vi "Handle Command.vi"(8 "error in (no error)":errorcluster, 9 "Data":variant, 10 "Command":string, 11 "RP100 in":refnum<class "RP100.lvclass">) -> (0 "error out":errorcluster, 1 "Processed Data":variant, 2 "Command":string, 3 "RP100 out":refnum<class "RP100.lvclass">)   [LabVIEW 2019, in "RP100.lvclass"]
uses:
  RP100.lvclass
  Typedefs/Output Channel--Enum.ctl
  Typedefs/Output State--Enum.ctl
  Typedefs/setStrain--Cluster.ctl
  RP100.lvclass/RP100.ctl
  Typedefs/setOutput--Cluster.ctl
  Typedefs/setLevel--Cluster.ctl
  Typedefs/getLevel--Cluster.ctl
  144ac86c-f3d3-4b89-933e-c91cd0042f1d.vi
  aaf9e925-0147-4d55-b975-571e4f63da02.vi
  6c0bf34a-ab55-4634-99ae-1a4930a83075.vi
  8b117c61-ef82-475d-98ae-2b78dab96990.vi
  <vilib>/JDP Science/JSONtext/JSON text to Variant.vi
  <vilib>/JDP Science/JSONtext/LVClass Serializer/JSONtext LVClass Serializer.lvclass
  <userlib>/LevyLab/Instrument Framework/Instrument Types/Strain/Instrument.Strain.lvclass
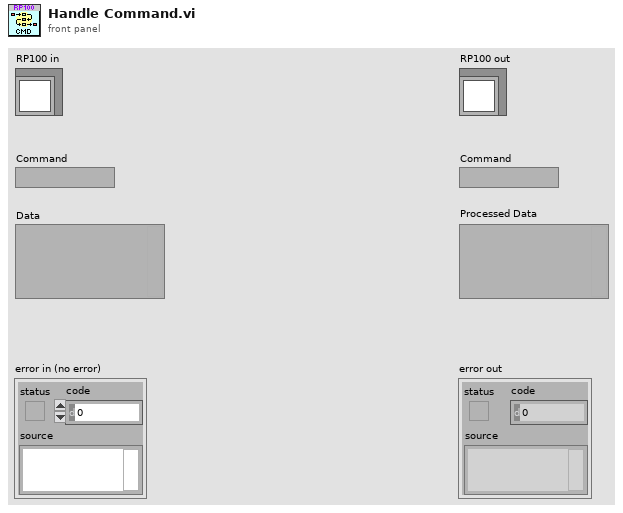
[diagram p1: front panel]
types:
  T1 = typedef "RP100.lvclass/setStrain--Cluster.ctl" = cluster{"Strain (V)":dbl, "Slew (V/s)":dbl}
  T2 = typedef "RP100.lvclass/Output Channel--Enum.ctl" = enum16{"Output 1", "Output 2"}
  T3 = typedef "RP100.lvclass/Output State--Enum.ctl" = enum16{"Shorted", "Enabled"}
  T4 = typedef "RP100.lvclass/setOutput--Cluster.ctl" = cluster{"State":T3}
  T5 = typedef "RP100.lvclass/setLevel--Cluster.ctl" = cluster{"Output Channel":T2, "Level (V)":dbl, "Slew (V/s)":dbl}
  T6 = typedef "RP100.lvclass/getLevel--Cluster.ctl" = cluster{"Channel":T2}
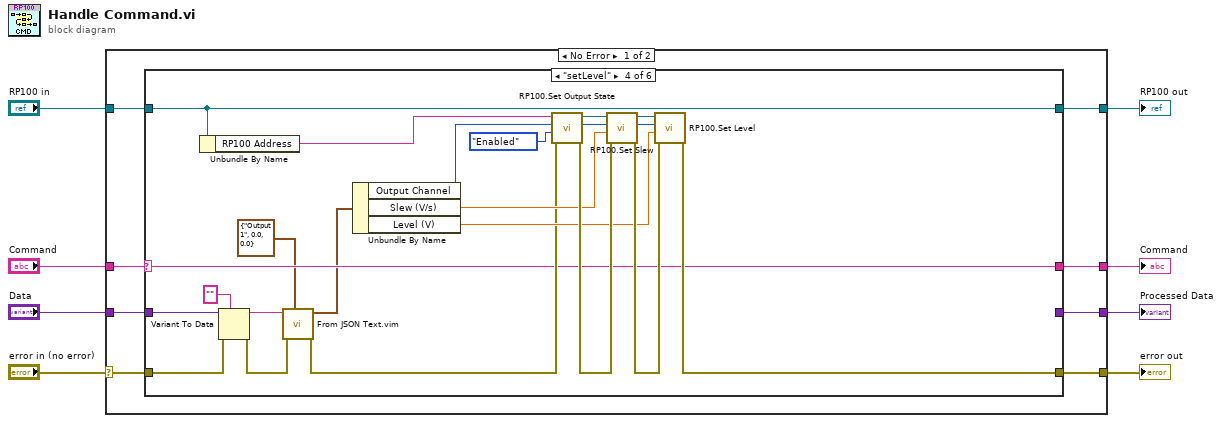
[diagram p0: block diagram]
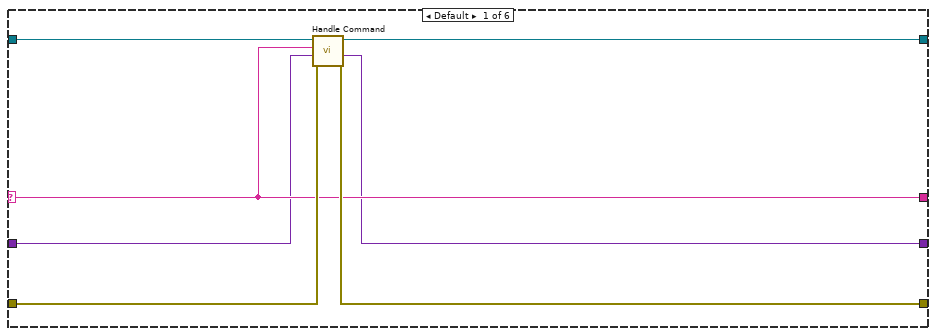
[diagram p2: hidden frame]
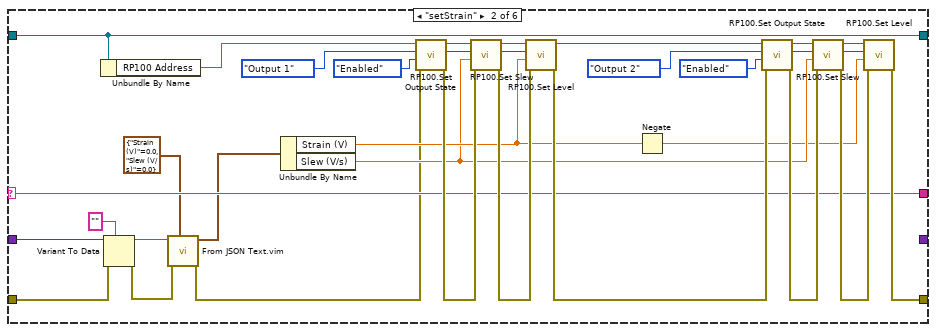
[diagram p3: hidden frame]
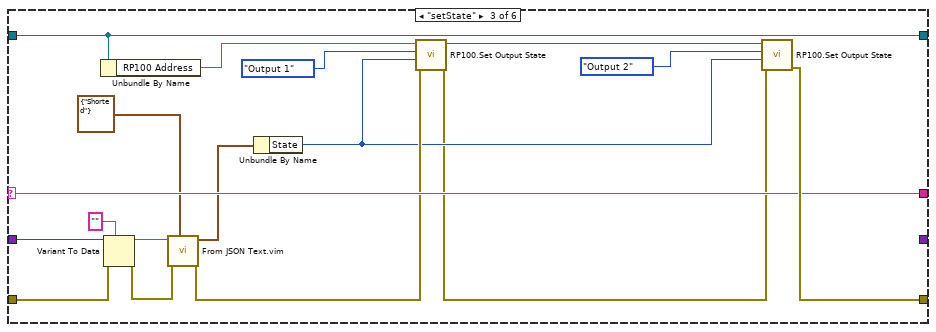
[diagram p4: hidden frame]
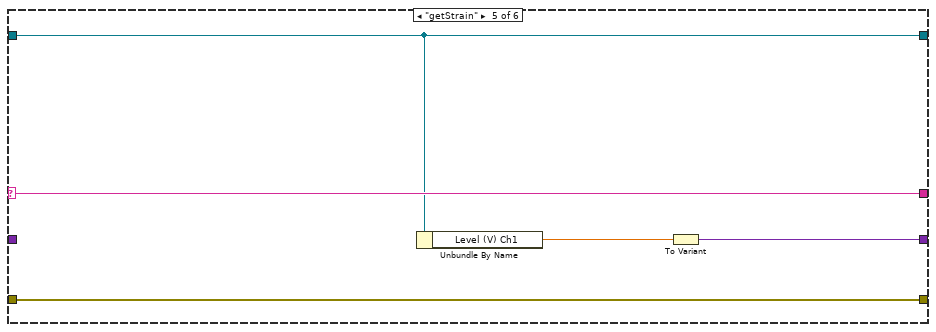
[diagram p5: hidden frame]
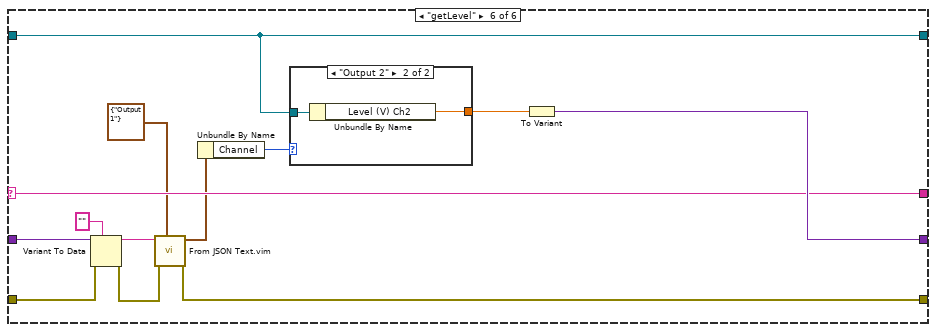
[diagram p6: hidden frame]
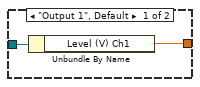
[diagram p7: hidden frame]
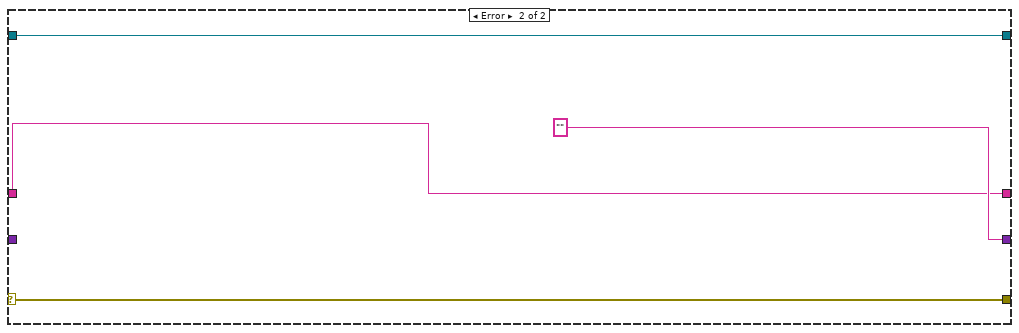
[diagram p8: hidden frame]
diagram:
  n1 = case shown="No Error" "error in (no error)" {
    selector: "error in (no error)" -> [w13 w121]
    tunnel: [w12 w121] -> w4
    tunnel: [w15 w120] -> w6
    tunnel: "RP100 in" -> [w16 w120]
    tunnel: "Command" -> [w10 w118]
    tunnel: [w14 "" ("error message (\"\")")] -> w3
    tunnel: [w11 w118] -> w2
    tunnel: "Data" -> [w9 _]
    frame No Error {
      n2 = case shown="\"setLevel\"" w10 {
        selector: w10 -> [w21 w35 w70 w80 w99 w109]
        tunnel: w16 -> [w20 w27 w64 w76 w96 w111]
        tunnel: [w19 w27 w64 w76 w96 w111] -> w15
        tunnel: [w17 _ _ _ w98 w113] -> w14
        tunnel: w13 -> [w23 w26 w63 w75 w100 w106]
        tunnel: [w22 w48 w71 w92 w100 w104] -> w12
        tunnel: [w21 w35 w70 w80 w99 w109] -> w11
        tunnel: w9 -> [w18 w32 w67 w82 _ w108]
        frame Default {
          n3 = call-parent "Handle Command.vi"("error in (no error)"=w23, "Data"=w18, "Command"=w21, "Instrument in"=w20) -> ("error out"=w22:errorcluster, "Processed Data"=w17:variant, "Instrument out"=w19:refnum<class "RP100.lvclass">)  [unwired: 4 in, 1 out]
        }
        frame "setStrain" {
          n4 = Unbundle By Name(w27) -> ("RP100 Address"=w25:string)
          n5 = Variant To Data(error in=w26, type="", Variant=w32) -> (data=w34:string, error out=w31:errorcluster)
          n6 = call "From JSON Text.vim"("Data Type and Default Value"=T1 {"Strain (V)"=0.0, "Slew (V/s)"=0.0} ("setStrain"), "error in (no error)"=w31, "JSON"=w34) -> ("error out"=w30:errorcluster, "Data out"=w24:T1)  [unwired: 7 in]
          n7 = Unbundle By Name(w24) -> ("Strain (V)"=w47:dbl, "Slew (V/s)"=w40:dbl)
          n8 = call "RP100.Set Output State.vi"("error in (no error)"=w30, "Output State"=Output_State--Enum."Enabled", "Output Channel"=Output_Channel--Enum."Output 1", "VISA resource name"=w25) -> ("error out"=w53:errorcluster, "Output Channel"=w45:T2, "VISA Refnum out"=w46:refnum<visa-resource-name>)  [unwired: 5 in]
          n9 = call "RP100.Set Slew.vi"("error in (no error)"=w53, "Slew (V/s)"=w40, "Output Channel"=w45, "VISA resource name"=w46) -> ("error out"=w52:errorcluster, "Output Channel"=w44:T2, "VISA Refnum out"=w43:refnum<visa-resource-name>)  [unwired: 5 in]
          n10 = call "RP100.Set Level.vi"("error in (no error)"=w52, "Level (V)"=w47, "Output Channel"=w44, "VISA resource name"=w43) -> ("error out"=w51:errorcluster, "VISA Refnum out"=w42:refnum<visa-resource-name>)  [unwired: 5 in, 1 out]
          n11 = Negate(x=w47) -> (-x=w39:dbl)
          n12 = call "RP100.Set Output State.vi"("error in (no error)"=w51, "Output State"=Output_State--Enum."Enabled", "Output Channel"=Output_Channel--Enum."Output 2", "VISA resource name"=w42) -> ("error out"=w50:errorcluster, "Output Channel"=w41:T2, "VISA Refnum out"=w36:refnum<visa-resource-name>)  [unwired: 5 in]
          n13 = call "RP100.Set Slew.vi"("error in (no error)"=w50, "Slew (V/s)"=w40, "Output Channel"=w41, "VISA resource name"=w36) -> ("error out"=w49:errorcluster, "Output Channel"=w38:T2, "VISA Refnum out"=w37:refnum<visa-resource-name>)  [unwired: 5 in]
          n14 = call "RP100.Set Level.vi"("error in (no error)"=w49, "Level (V)"=w39, "Output Channel"=w38, "VISA resource name"=w37) -> ("error out"=w48:errorcluster)  [unwired: 5 in, 2 out]
        }
        frame "setState" {
          n15 = Unbundle By Name(w64) -> ("RP100 Address"=w62:string)
          n16 = Variant To Data(error in=w63, type="", Variant=w67) -> (data=w69:string, error out=w66:errorcluster)
          n17 = call "From JSON Text.vim"("Data Type and Default Value"=T4 {"State"=enum."Shorted"} ("setOutput"), "error in (no error)"=w66, "JSON"=w69) -> ("error out"=w65:errorcluster, "Data out"=w61:T4)  [unwired: 7 in]
          n18 = Unbundle By Name(w61) -> ("State"=w59:T3)
          n19 = call "RP100.Set Output State.vi"("error in (no error)"=w65, "Output State"=w59, "Output Channel"=Output_Channel--Enum."Output 1", "VISA resource name"=w62) -> ("error out"=w57:errorcluster, "VISA Refnum out"=w58:refnum<visa-resource-name>)  [unwired: 5 in, 1 out]
          n20 = call "RP100.Set Output State.vi"("error in (no error)"=w57, "Output State"=w59, "Output Channel"=Output_Channel--Enum."Output 2", "VISA resource name"=w58) -> ("error out"=w71:errorcluster)  [unwired: 5 in, 2 out]
        }
        frame "setLevel" {
          n21 = Unbundle By Name(w76) -> ("RP100 Address"=w74:string)
          n22 = Variant To Data(error in=w75, type="", Variant=w82) -> (data=w84:string, error out=w78:errorcluster)
          n23 = call "From JSON Text.vim"("Data Type and Default Value"=T5 {"Output Channel"=enum."Output 1", "Level (V)"=0.0, "Slew (V/s)"=0.0} ("setLevel"), "error in (no error)"=w78, "JSON"=w84) -> ("error out"=w81:errorcluster, "Data out"=w77:T5)  [unwired: 7 in]
          n24 = Unbundle By Name(w77) -> ("Output Channel"=w86:T2, "Slew (V/s)"=w87:dbl, "Level (V)"=w85:dbl)
          n25 = call "RP100.Set Output State.vi"("error in (no error)"=w81, "Output State"=Output_State--Enum."Enabled", "Output Channel"=w86, "VISA resource name"=w74) -> ("error out"=w94:errorcluster, "Output Channel"=w90:T2, "VISA Refnum out"=w91:refnum<visa-resource-name>)  [unwired: 5 in]
          n26 = call "RP100.Set Slew.vi"("error in (no error)"=w94, "Slew (V/s)"=w87, "Output Channel"=w90, "VISA resource name"=w91) -> ("error out"=w93:errorcluster, "Output Channel"=w89:T2, "VISA Refnum out"=w88:refnum<visa-resource-name>)  [unwired: 5 in]
          n27 = call "RP100.Set Level.vi"("error in (no error)"=w93, "Level (V)"=w85, "Output Channel"=w89, "VISA resource name"=w88) -> ("error out"=w92:errorcluster)  [unwired: 5 in, 2 out]
        }
        frame "getStrain" {
          n28 = Unbundle By Name(w96) -> ("Level (V) Ch1"=w97:dbl)
          n29 = To Variant(anything=w97) -> (Variant=w98:variant)
        }
        frame "getLevel" {
          n30 = Variant To Data(error in=w106, type="", Variant=w108) -> (data=w110:string, error out=w105:errorcluster)
          n31 = call "From JSON Text.vim"("Data Type and Default Value"=T6 {"Channel"=enum."Output 1"} ("getLevel"), "error in (no error)"=w105, "JSON"=w110) -> ("error out"=w104:errorcluster, "Data out"=w103:T6)  [unwired: 7 in]
          n32 = Unbundle By Name(w103) -> ("Channel"=w102:T2)
          n33 = case shown="\"Output 2\"" w102 {
            tunnel: [w115 w117] -> w112
            tunnel: w111 -> [w114 w116]
            frame "Output 1", Default {
              n34 = Unbundle By Name(w114) -> ("Level (V) Ch1"=w115:dbl)
            }
            frame "Output 2" {
              n35 = Unbundle By Name(w116) -> ("Level (V) Ch2"=w117:dbl)
            }
          }
          n36 = To Variant(anything=w112) -> (Variant=w113:variant)
        }
      }
    }
    frame Error {
    }
  }
  "error out" <- w4
  "RP100 out" <- w6
  "Processed Data" <- w3
  "Command" <- w2
